vi "Get all existing alisases.vi"() -> (3 "Existing Aliases":string[](array[string]))   [LabVIEW 2013]
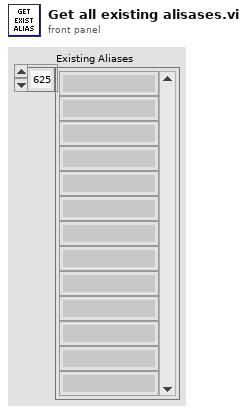
[diagram p1: front panel]
types:
  T1 = typedef "mysql_authentication.ctl" = cluster{"User":string, "Password":string, "Database":string}
  T2 = cluster{"Port":u16, "IP Address":string, "Authentication":T1}
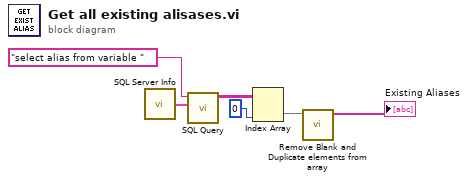
[diagram p0: block diagram]
diagram:
  n1 = call "SQL Server Info.vi"() -> ("SQL Server Info"=w6:T2)
  n2 = call "SQL Query.vi"("SQL Server Info"=w6, "Query"="select alias from variable ") -> ("data"=w5:string[][])  [unwired: 8 in, 1 out]
  n3 = Index Array(array=w5, index (col)=0 ("disabled index (col)")) -> (element=w2:string[])  [unwired: 1 in]
  n4 = call "Remove Blank and Duplicate elements from array.vi"("IP Addresses"=w2) -> ("String out"=→"Existing Aliases":string[])  [unwired: 10 in]
